vi "Konwersja to dig.vi"() -> ()   [LabVIEW 2013]
uses:
  <vilib>/Waveform/DWDTOps.llb/Digital Pattern Generator (Random).vi
  <vilib>/Waveform/DWDTOps.llb/DWDT Boolean Array to Digital.vi
panel:
  out "values":string
  out "size(s) 2":i32
  out "size(s)":i32
  out "dt":dbl
  out "Mixed Signal Graph":T1(graph)
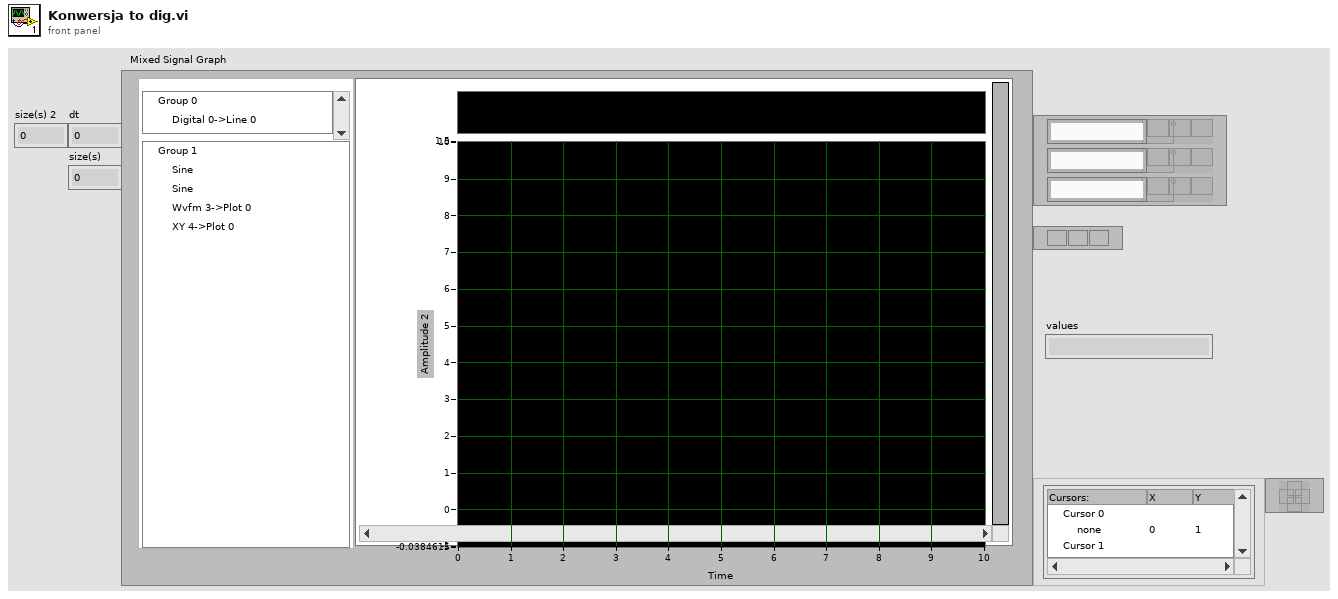
[diagram p1: front panel]
types:
  T1 = cluster{"digital waveform":digitalwaveform, "Waveform":waveform(dbl), "Sine":dynamicdata, dbl[], cluster{dbl[], dbl[]}}
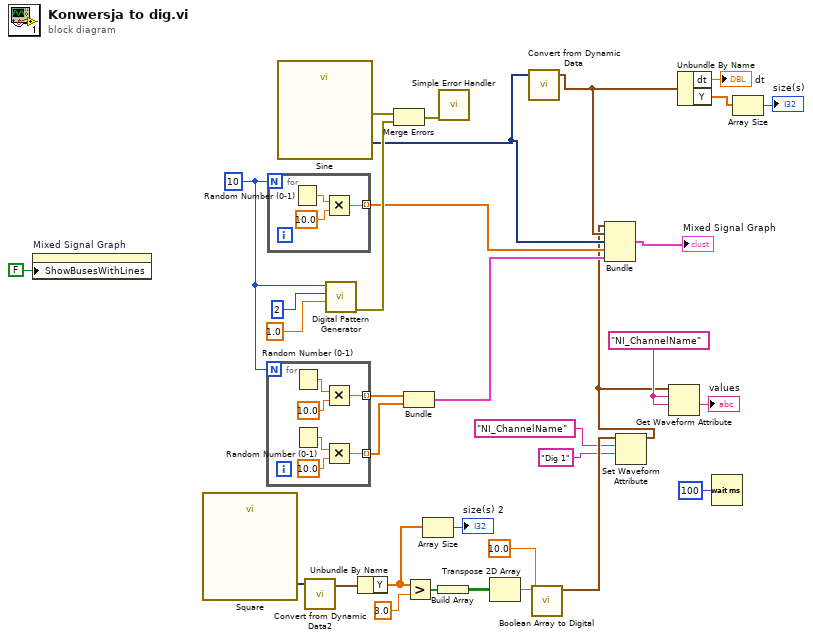
[diagram p0: block diagram]
diagram:
  w8 = "NI_ChannelName" ("name")
  w30 = 10
  n1 = property on="Mixed Signal Graph" class="MixedGraph (strict)"("ShowBusesWithLines"=FALSE ("Show Buses With Lines")) -> ()  [unwired: 2 in, 2 out]
  n2 = call "Square"() -> ("Square"=w18:dynamicdata)  [unwired: 14 in, 1 out]
  n3 = for {
    N: w30 -> [_]
    tunnel: [w38] -> w28 mode=indexing
    tunnel: [w34] -> w29 mode=indexing
    n4 = Random Number (0-1)() -> (number: 0 to 1=w39:dbl)
    n5 = Random Number (0-1)() -> (number: 0 to 1=w35:dbl)
    n6 = Multiply(x=w39, y=10.0) -> (x*y=w38:dbl)
    n7 = Multiply(x=w35, y=10.0) -> (x*y=w34:dbl)
  }
  n8 = for {
    N: w30 -> [_]
    tunnel: [w41] -> w25 mode=indexing
    n9 = Random Number (0-1)() -> (number: 0 to 1=w42:dbl)
    n10 = Multiply(x=w42, y=10.0) -> (x*y=w41:dbl)
  }
  n11 = call "Sine"() -> ("Sine"=w23:dynamicdata, "error out"=w31:errorcluster)  [unwired: 14 in]
  n12 = call "Convert from Dynamic Data2"("Dynamic Data Type"=w18) -> ("Waveform"=w17:waveform(dbl))  [unwired: 3 in]
  n13 = call-poly <vilib>:"Digital Pattern Generator.vi"("sample rate"=1.0, "number of signals"=u32 2, "number of samples"=w30) -> ("error out"=w32:errorcluster)  [unwired: 7 in, 1 out]
  n14 = Unbundle By Name(w17) -> ("Y"=w11:dbl[])
  n15 = Merge Errors(w31, w32) -> (w33:errorcluster)
  n16 = Bundle(w28, w29) -> (w24:cluster{dbl[], dbl[]})  [unwired: 1 in]
  n17 = Greater?(x=w11, y=3.0) -> (0:w15:bool[])
  n18 = Array Size(array=w11) -> (size(s)=→"size(s) 2":i32)
  n19 = Build Array(w15) -> (w13:bool[][])
  n20 = call <vilib>:"Simple Error Handler.vi"("error in (no error)"=w33) -> ()  [unwired: 4 in, 5 out]
  n21 = Transpose 2D Array(2D array=w13) -> (transposed array=w12:bool[][])
  n22 = call "Convert from Dynamic Data"("Dynamic Data Type"=w23) -> ("Waveform"=w6:waveform(dbl))  [unwired: 3 in]
  n23 = call-poly <vilib>:"Boolean Array to Digital.vi"("sample rate"=10.0, "boolean array"=w12) -> ("digital waveform"=w5:digitalwaveform)  [unwired: 8 in, 1 out]
  n24 = Set Waveform Attribute(5:"Dig 1" ("name"), 6:"NI_ChannelName" ("name"), 7:w5) -> (3:w2:digitalwaveform)  [unwired: 1 in, 2 out]
  n25 = Bundle("digital waveform"=w2, "Waveform"=w6, "Sine"=w23, w25, w24) -> (→"Mixed Signal Graph":T1)  [unwired: 1 in]
  n26 = Get Waveform Attribute(5:w8, 6:w8, 7:w2) -> (1:→"values":string)  [unwired: 1 in, 3 out]
  n27 = Unbundle By Name(w6) -> ("dt"=→"dt":dbl, "Y"=w21:dbl[])
  n28 = Wait (ms)(milliseconds to wait=u32 100) -> ()  [unwired: 1 out]
  n29 = Array Size(array=w21) -> (size(s)=→"size(s)":i32)
